vi "Generate Filepath.vi"(8 "error in":errorcluster, 11 "Log in":refnum<class "Log.lvclass">) -> (0 "error out":errorcluster, 3 "Log out":refnum<class "Log.lvclass">)   [LabVIEW 2017, in "Report_lib.lvlib" / "Log.lvclass"]
doc: "ThisSubVI generate full filepath\nfor create external file"
uses:
  Log.lvclass
  Log.lvclass/Log.ctl
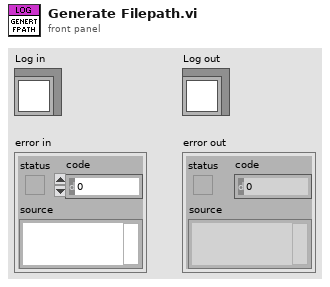
[diagram p1: front panel]
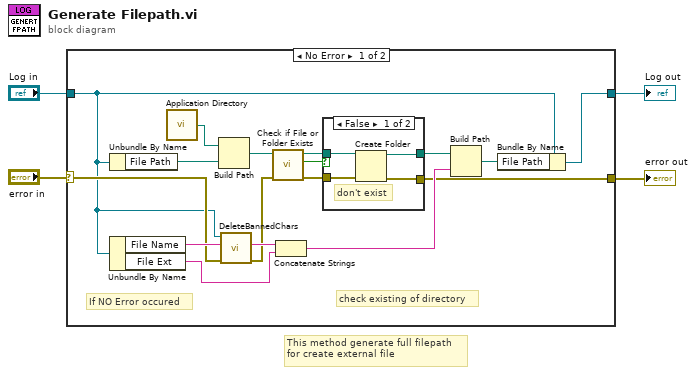
[diagram p0: block diagram]
diagram:
  # "This method generate full filepath\nfor create external file"
  n1 = case shown="No Error" "error in" {
    selector: "error in" -> [w8 w29]
    tunnel: [w13 w29] -> w3
    tunnel: [w11 w28] -> w1
    tunnel: "Log in" -> [w6 w28]
    frame No Error {
      # "If NO Error occured"
      # "check existing of directory"
      n2 = Unbundle By Name(w6) -> ("File Path"=w5:path)
      n3 = Unbundle By Name(w6) -> ("File Name"=w10:string, "File Ext"=w16:string)
      n4 = call <vilib>:"Application Directory.vi"() -> ("Application Directory"=w17:path)
      n5 = Build Path(base path=w17, name or relative path=w5) -> (appended path=w21:path)
      n6 = call "DeleteBannedChars.vi"("error in"=w8, "string in"=w10, "Log in"=w6) -> ("error out"=w7:errorcluster, "string out"=w9:string)  [unwired: 6 in, 1 out]
      n7 = call <vilib>:"Check if File or Folder Exists.vi"("error in (no error)"=w7, "path"=w21) -> ("error out"=w20:errorcluster, "file or folder exists?"=w18:bool, "dup path"=w19:path)  [unwired: 7 in]
      n8 = Concatenate Strings(w9, w16) -> (w15:string)
      n9 = case shown="False" w18 {
        tunnel: w19 -> [w25 w27]
        tunnel: [w23 w27] -> w14
        tunnel: w20 -> [w24 w26]
        tunnel: [w22 w26] -> w13
        frame False {
          # "don't exist"
          n10 = Create Folder(path (use dialog)=w25, error in=w24) -> (created path=w23:path, error out=w22:errorcluster)  [unwired: 1 in, 1 out]
        }
        frame True {
          # "exist"
        }
      }
      n11 = Build Path(base path=w14, name or relative path=w15) -> (appended path=w12:path)
      n12 = Bundle By Name(cluster=w6, "File Path"=w12) -> (w11:refnum<class "Log.lvclass">)
    }
    frame Error {
    }
  }
  "error out" <- w3
  "Log out" <- w1
